vi "build_queue.vi"(8 "Scan settings array":T2[](array[typedef]) {"Settling delay (s)" min=0.0; "J-t illumination" items=["Light only", "Dark only", "Light then dark", "Dark then light"]; "Measurement speed" items=["Fast", "Normal", "High accuracy"]; "Illumination" items=["Light only", "Dark only", "Light then dark", "Dark then light"]; "Only repeat for best pixel" items=["only for best pixel", "for best 2 pixels", "for best 3 pixels", "for best 4 pixels", "for best 5 pixels", "for best 6 pixels", "for best 7 pixels", "for all pixels"]; "No. of repeat scans" min=1.0 step=1.0; "Max power best pixel only" items=["only the best pixel", "the best 2 pixels", "the best 3 pixels", "the best 4 pixels", "the best 5 pixels", "the best 6 pixels", "the best 7 pixels", "all pixels"]; "J-t best pixel only" items=["only the best pixel", "the best 2 pixels", "the best 3 pixels", "the best 4 pixels", "the best 5 pixels", "the best 6 pixels", "the best 7 pixels", "all pixels"]; "J-t measurement speed" items=["Fast", "Normal", "High Accuracy"]; "Stabilisation mode" items=["V", "I"]; "Measurement delay (s)" min=0.01}, 11 "Device details":T1={"Cell Position"=1, "Cell Label"="", "Pixel to measure"=0, "Area (cm^2)"=0.0919, "Variable"="", "Variable value"="", "Scan settings"=0} {"Scan settings" items=["Default_inv", "Default_std"]; "Pixel to measure" items=["All", "1", "2", "3", "4", "5", "6", "7", "8"]}) -> (3 "Measurement queue":T3(array[cluster]) {"Pixel to measure" items=["All", "1", "2", "3", "4", "5", "6", "7", "8"]})   [LabVIEW 2016]
uses:
  TypeDefs/scan_settings.ctl
panel:
  out "Max power best pixel only":u16
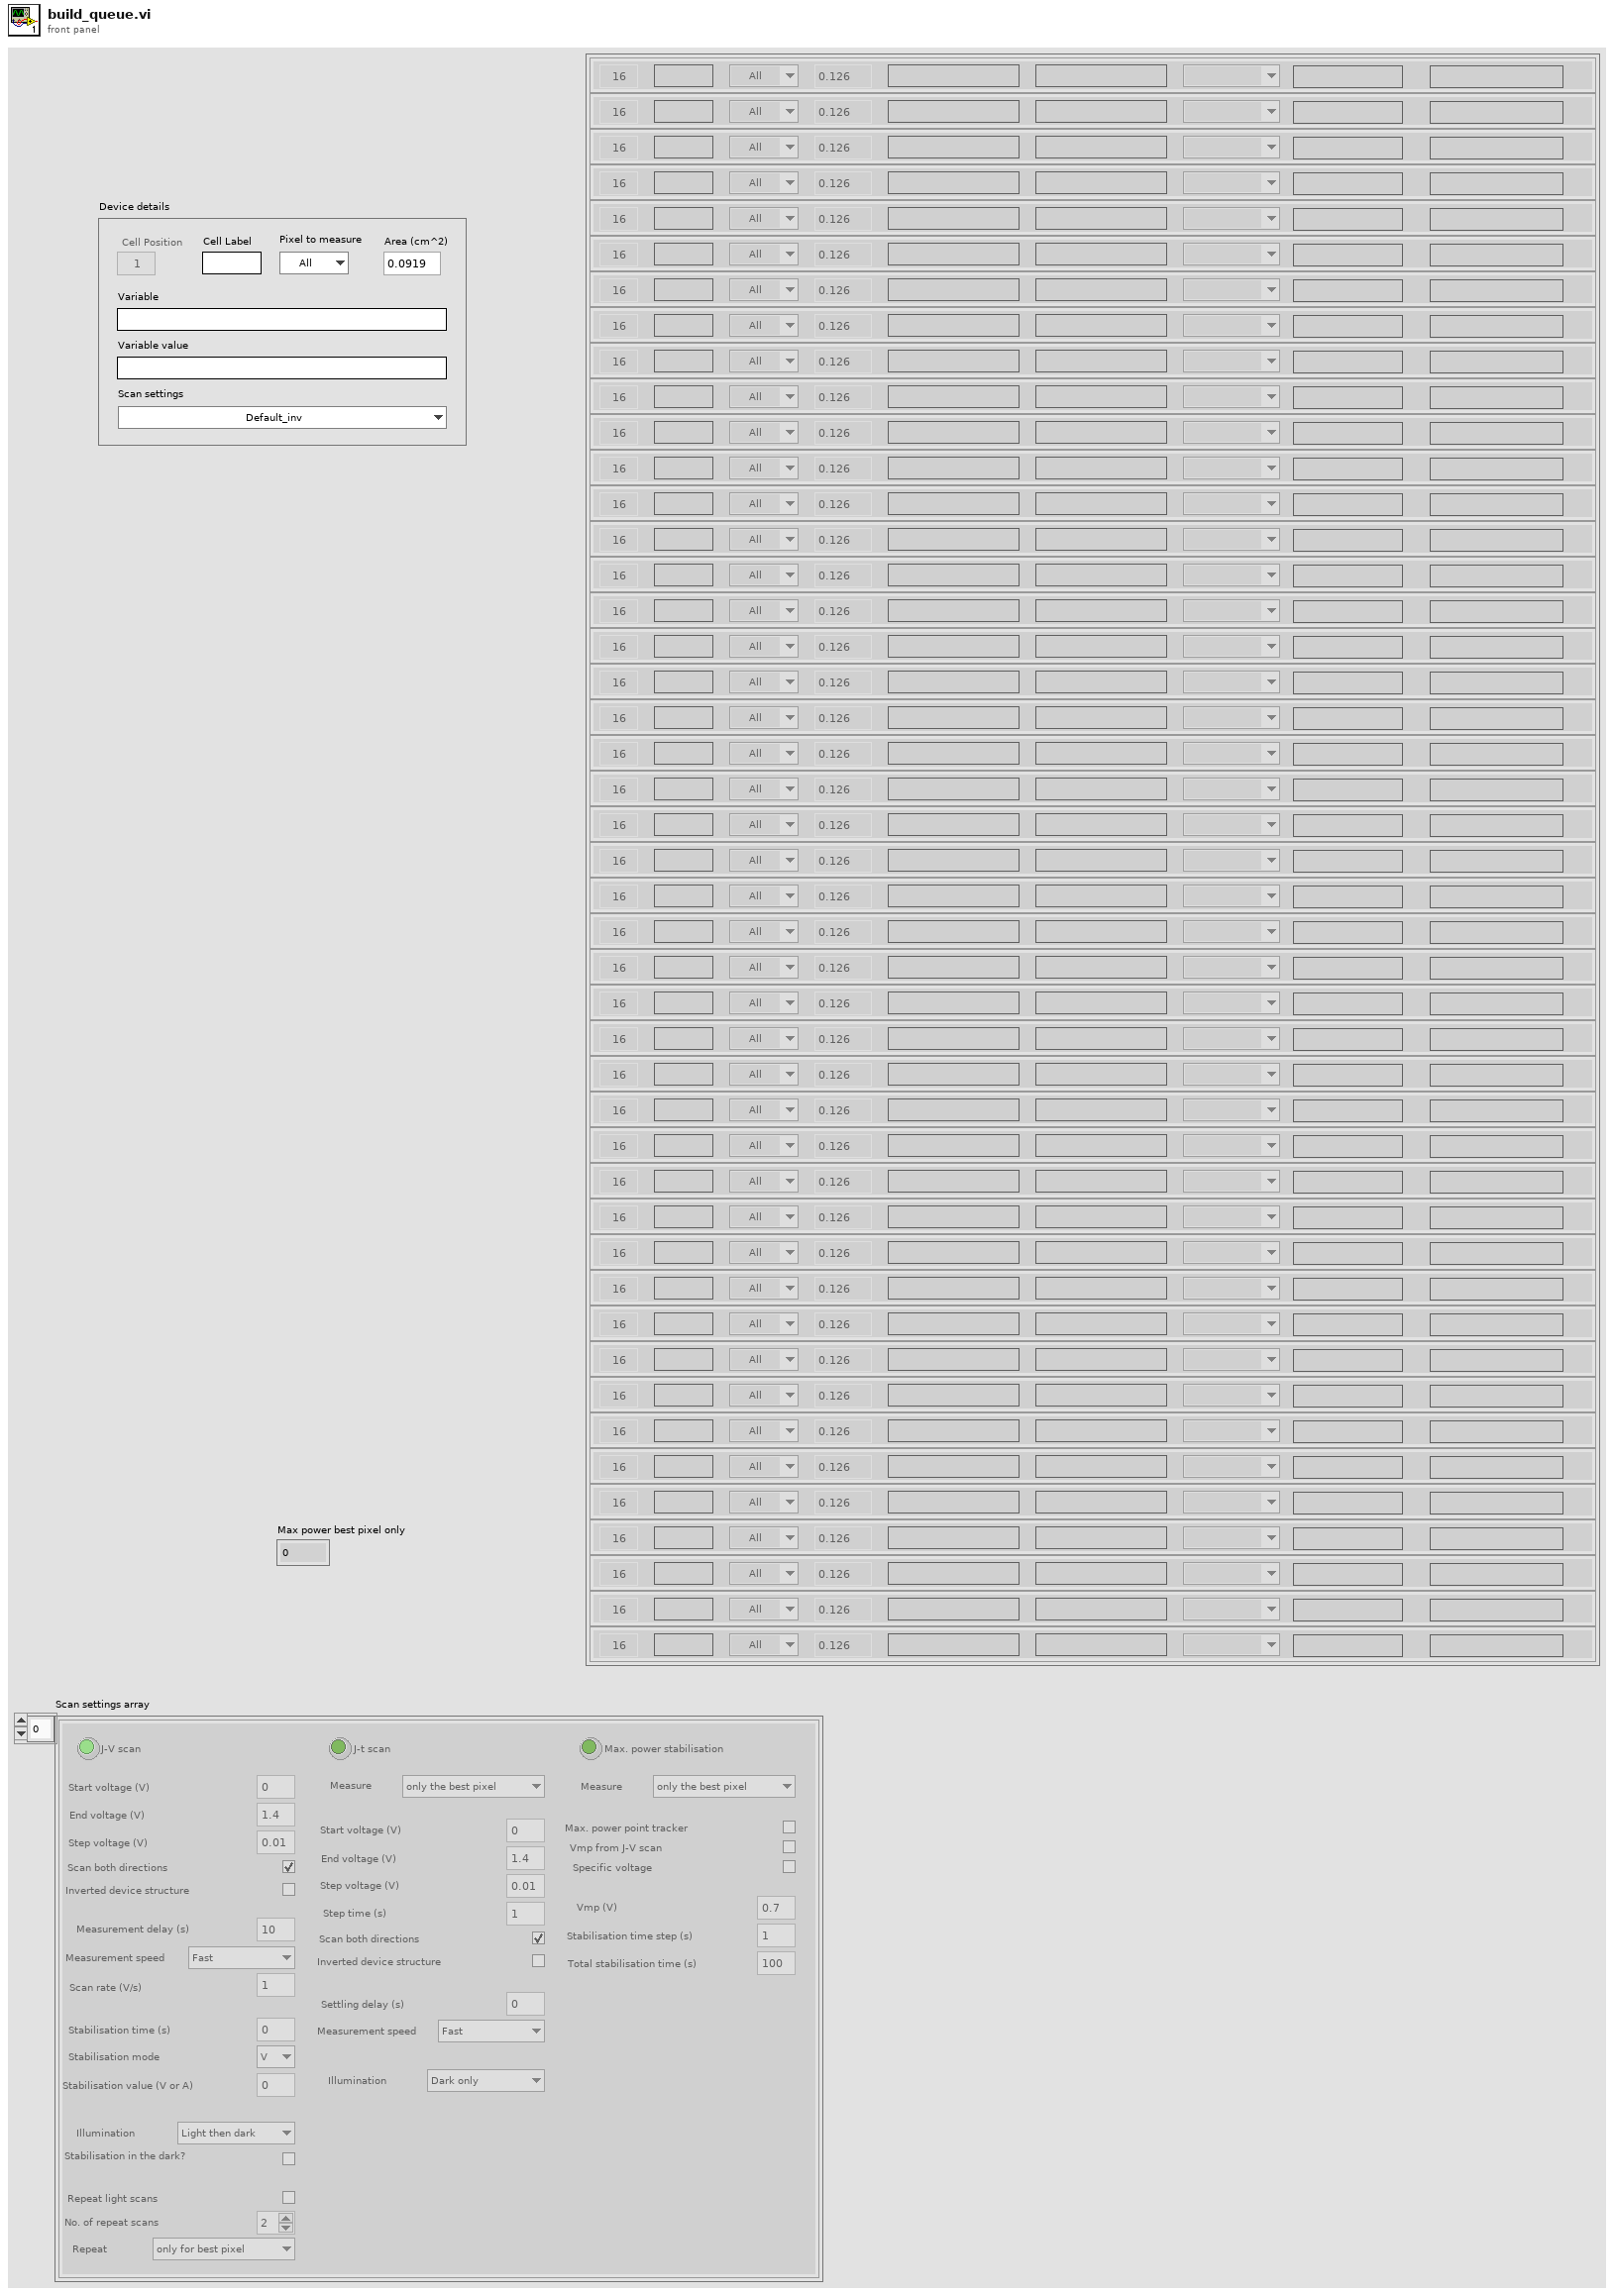
[diagram p1: front panel]
types:
  T1 = cluster{"Cell Position":i32, "Cell Label":string, "Pixel to measure":u16, "Area (cm^2)":dbl, "Variable":string, "Variable value":string, "Scan settings":u16}
  T2 = typedef "scan_settings.ctl" = cluster{"J-V scan":bool, "Start voltage (V)":dbl, "End voltage (V)":dbl, "Step voltage (V)":dbl, "Scan both directions":bool, "Inverted device structure":bool, "Measurement delay (s)":dbl, "Measurement speed":u8, "Scan rate (V/s)":dbl, "Stabilisation time (s)":dbl, "Stabilisation mode":u16, "Stabilisation value (V or A) ":dbl, "Illumination":u16, "Stabilisation in the dark?":bool, "Repeat light scans":bool, "No. of repeat scans":dbl, "Only repeat for best pixel":u16, "J-t scan":bool, "J-t best pixel only":u16, "J-t start voltage (V)":dbl, "J-t end voltage (V)":dbl, "J-t step voltage (V)":dbl, "Step time (s)":dbl, "J-t scan both directions":bool, "J-t inverted device structure":bool, "Settling delay (s)":dbl, "J-t measurement speed":u16, "J-t illumination":u16, "Max. power stabilisation":bool, "Max power best pixel only":u16, "Max. power point tracker":bool, "Vmp from J-V scan":bool, "Max P stab. Specific voltage":bool, "Vmp (V)":dbl, "Stabilisation time step (s)":dbl, "Total stabilisation time (s)":dbl}
  T3 = cluster{"Cell Position":i32, "Cell Label":string, "Pixel to measure":u16, "Area (cm^2)":dbl, "Variable":string, "Variable value":string, "Scan settings in queue":u16, "Light or dark":string, "Measurement type":string}[]
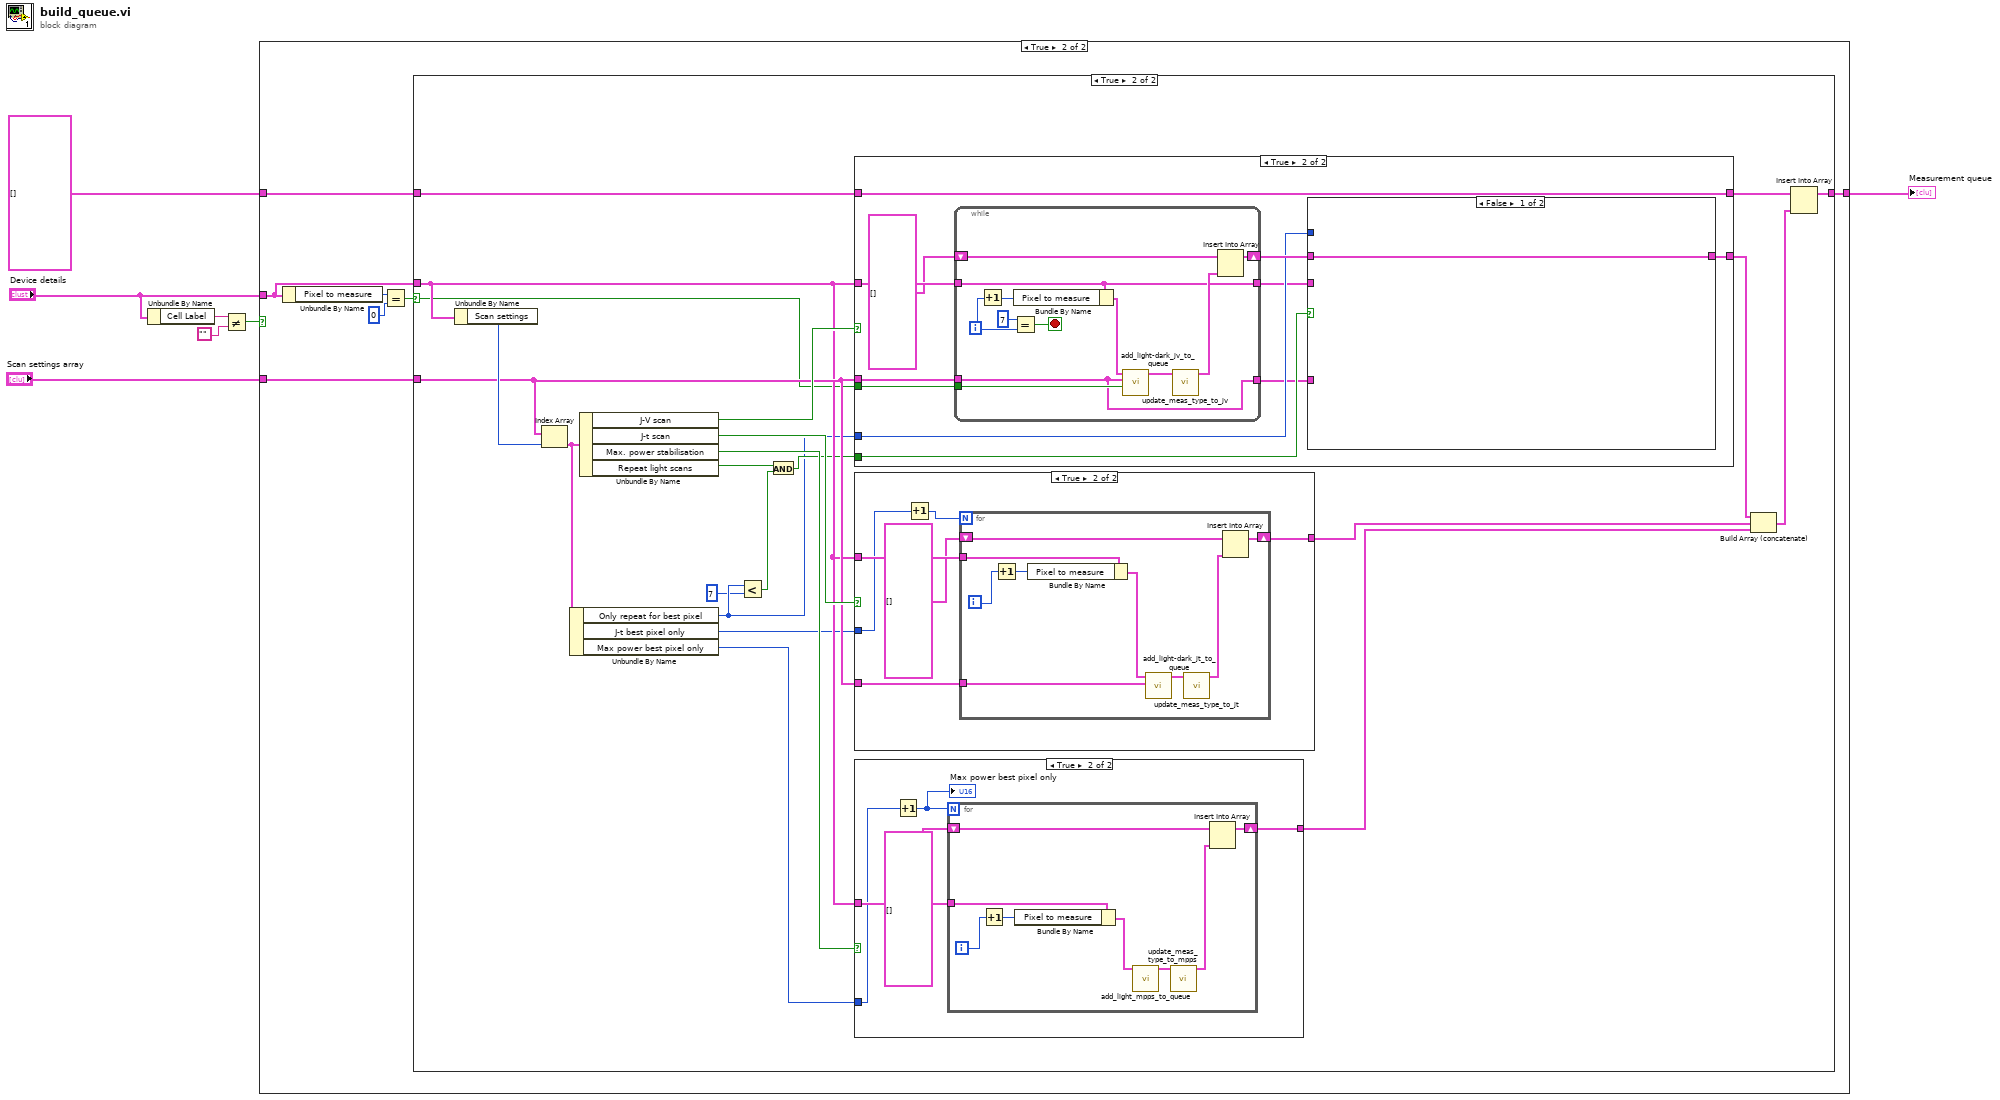
[diagram p0: block diagram]
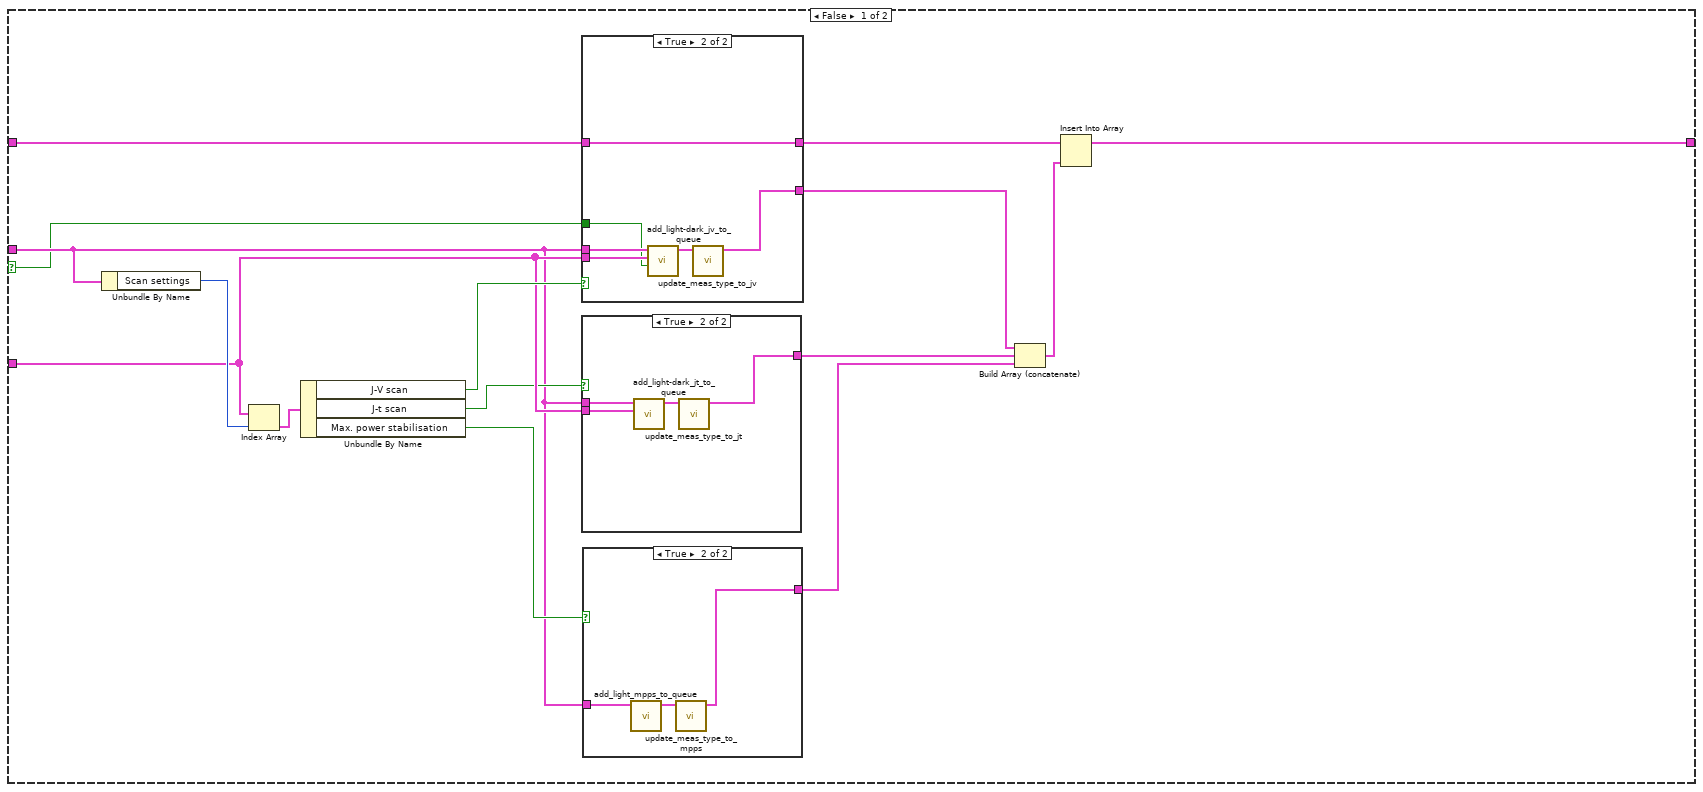
[diagram p3: hidden frame]
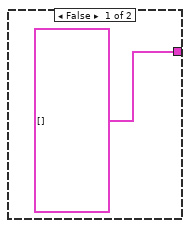
[diagram p4: hidden frame]
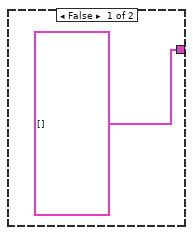
[diagram p5: hidden frame]
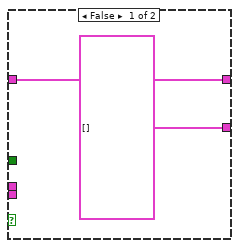
[diagram p6: hidden frame]
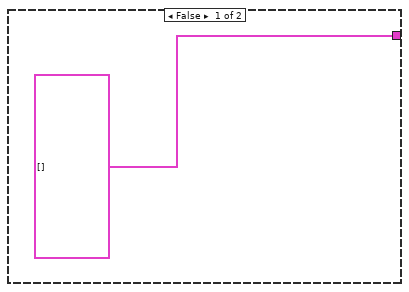
[diagram p7: hidden frame]
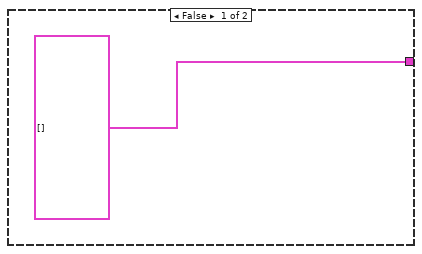
[diagram p8: hidden frame]
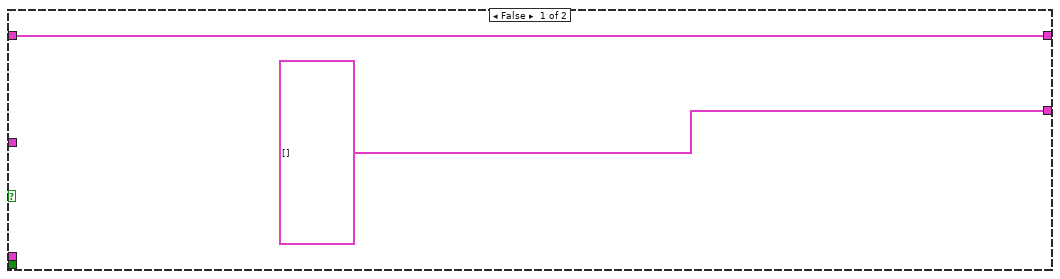
[diagram p9: hidden frame]
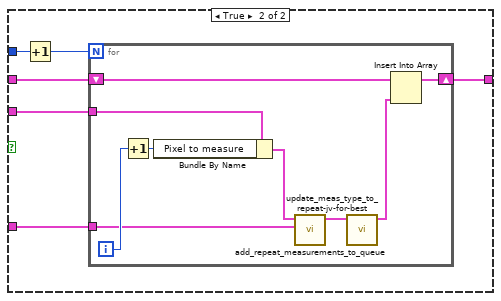
[diagram p10: hidden frame]
diagram:
  n1 = Unbundle By Name("Device details") -> ("Cell Label"=w3:string)
  n2 = Not Equal?(x=w3, y="") -> (x != y?=w1:bool)
  n3 = case shown="True" w1 {
    tunnel: [w8 w12] -> w6
    tunnel: "Device details" -> [_ w11]
    tunnel: T3 [] ("Measurement queue") -> [w8 w10]
    tunnel: "Scan settings array" -> [_ w9]
    frame False {
    }
    frame True {
      n4 = Unbundle By Name(w11) -> ("Pixel to measure"=w15:u16)
      n5 = Equal?(x=w15, y=0) -> (x = y?=w13:bool)
      n6 = case shown="True" w13 {
        selector: w13 -> [w16 w53]
        tunnel: w11 -> [w19 w60]
        tunnel: [w30 w67] -> w12
        tunnel: w10 -> [w20 w59]
        tunnel: w9 -> [w26 w63]
        frame False {
          n7 = Unbundle By Name(w19) -> ("Scan settings"=w29:u16)
          n8 = Index Array(array=w26, index=w29) -> (element=w18:T2)
          n9 = Unbundle By Name(w18) -> ("J-V scan"=w27:bool, "J-t scan"=w25:bool, "Max. power stabilisation"=w21:bool)
          n10 = case shown="True" w27 {
            tunnel: w19 -> [_ w46]
            tunnel: w26 -> [_ w45]
            tunnel: [w41 w44] -> w28
            tunnel: w20 -> [w41 w44]
            tunnel: [T3 [] ("Measurement queue") w43] -> w17
            tunnel: w16 -> [_ w42]
            frame False {
            }
            frame True {
              n11 = call "add_light-dark_jv_to_queue.vi"("Measuring all pixels on cell?"=w42, "Scan settings array"=w45, "Cell settings cluster"=w46) -> ("Light/dark array"=w47:T3)  [unwired: 8 in]
              n12 = call "update_meas_type_to_jv.vi"("Cell details array in"=w47) -> ("Cell details array out"=w43:T3)  [unwired: 10 in]
            }
          }
          n13 = case shown="True" w25 {
            tunnel: w19 -> [_ w38]
            tunnel: w26 -> [_ w37]
            tunnel: [T3 [] ("Measurement queue") w36] -> w24
            frame False {
            }
            frame True {
              n14 = call "add_light-dark_jt_to_queue.vi"("Scan settings array"=w37, "Cell settings cluster"=w38) -> ("Light/dark array"=w39:T3)  [unwired: 9 in]
              n15 = call "update_meas_type_to_jt.vi"("Cell details array in"=w39) -> ("Cell details array out"=w36:T3)  [unwired: 10 in]
            }
          }
          n16 = case shown="True" w21 {
            tunnel: [T3 [] ("Measurement queue") w32] -> w23
            tunnel: w19 -> [_ w33]
            frame False {
            }
            frame True {
              n17 = call "add_light_mpps_to_queue.vi"("Cell settings cluster"=w33) -> ("Light/dark array"=w34:T3)  [unwired: 10 in]
              n18 = call "update_meas_type_to_mpps.vi"("Cell details array in"=w34) -> ("Cell details array out"=w32:T3)  [unwired: 10 in]
            }
          }
          n19 = Build Array (concatenate)(w17, w24, w23) -> (w22:T3)
          n20 = Insert Into Array(array=w28, new element=w22) -> (w30:T3)  [unwired: 1 in]
        }
        frame True {
          n21 = Unbundle By Name(w60) -> ("Scan settings"=w69:u16)
          n22 = Index Array(array=w63, index=w69) -> (element=w56:T2)
          n23 = Unbundle By Name(w56) -> ("Only repeat for best pixel"=w49:u16, "J-t best pixel only"=w55:u16, "Max power best pixel only"=w54:u16)
          n24 = Unbundle By Name(w56) -> ("J-V scan"=w68:bool, "J-t scan"=w64:bool, "Max. power stabilisation"=w62:bool, "Repeat light scans"=w52:bool)
          n25 = Less?(x=w49, y=u16 7 ("x")) -> (x < y?=w51:bool)
          n26 = And(x=w52, y=w51) -> (x .and. y?=w50:bool)
          n27 = case shown="True" w68 {
            tunnel: [w101 w110] -> w58
            tunnel: w59 -> [w101 w110]
            tunnel: w60 -> [_ w112]
            tunnel: w63 -> [_ w111]
            tunnel: [T3 [] ("Measurement queue") w108] -> w57
            tunnel: w53 -> [_ w109]
            tunnel: w50 -> [_ w106]
            tunnel: w49 -> [_ w105]
            frame False {
            }
            frame True {
              n28 = while {
                tunnel: w112 -> [w114]
                shift-right: [w120] -> w107
                shift-left: T3 [] ("Measurement queue") -> [w119]
                tunnel: w111 -> [w113]
                tunnel: w109 -> [w115]
                tunnel: [w114] -> w104
                tunnel: [w113] -> w103
                i -> [w122]
                stop <- w124 stop-if-true
                n29 = Increment(x=w122) -> (x+1=w123:i32)
                n30 = Equal?(x=7, y=w122) -> (x = y?=w124:bool)
                n31 = Bundle By Name(cluster=w114, "Pixel to measure"=w123) -> (w118:T1)
                n32 = call "add_light-dark_jv_to_queue.vi"("Measuring all pixels on cell?"=w115, "Scan settings array"=w113, "Cell settings cluster"=w118) -> ("Light/dark array"=w117:T3)  [unwired: 8 in]
                n33 = call "update_meas_type_to_jv.vi"("Cell details array in"=w117) -> ("Cell details array out"=w116:T3)  [unwired: 10 in]
                n34 = Insert Into Array(array=w119, new element=w116) -> (w120:T3)  [unwired: 1 in]
              }
              n35 = case shown="False" w106 {
                tunnel: [w125 w130] -> w108
                tunnel: w107 -> [w125 w131]
                tunnel: w105 -> [_ w127]
                tunnel: w104 -> [_ w129]
                tunnel: w103 -> [_ w128]
                frame False {
                }
                frame True {
                  n36 = Increment(x=w127) -> (x+1=w126:u16)
                  n37 = for {
                    N: w126 -> [_]
                    shift-right: [w139] -> w130
                    shift-left: w131 -> [w140]
                    tunnel: w129 -> [w134]
                    tunnel: w128 -> [w133]
                    i -> [w138]
                    n38 = Increment(x=w138) -> (x+1=w137:i32)
                    n39 = Bundle By Name(cluster=w134, "Pixel to measure"=w137) -> (w136:T1)
                    n40 = call "add_repeat_measurements_to_queue.vi"("Scan settings array"=w133, "Cell settings cluster"=w136) -> ("Repeat light array"=w135:T3)  [unwired: 9 in]
                    n41 = call "update_meas_type_to_repeat-jv-for-best.vi"("Cell details array in"=w135) -> ("Cell details array out"=w132:T3)  [unwired: 10 in]
                    n42 = Insert Into Array(array=w140, new element=w132) -> (w139:T3)  [unwired: 1 in]
                  }
                }
              }
            }
          }
          n43 = case shown="True" w64 {
            tunnel: [T3 [] ("Measurement queue") w90] -> w65
            tunnel: w60 -> [_ w89]
            tunnel: w63 -> [_ w88]
            tunnel: w55 -> [_ w85]
            frame False {
            }
            frame True {
              n44 = Increment(x=w85) -> (x+1=w86:u16)
              n45 = for {
                N: w86 -> [_]
                tunnel: w89 -> [w97]
                shift-right: [w96] -> w90
                shift-left: T3 [] ("Measurement queue") -> [w95]
                tunnel: w88 -> [w93]
                i -> [w98]
                n46 = Increment(x=w98) -> (x+1=w99:i32)
                n47 = Bundle By Name(cluster=w97, "Pixel to measure"=w99) -> (w94:T1)
                n48 = call "add_light-dark_jt_to_queue.vi"("Scan settings array"=w93, "Cell settings cluster"=w94) -> ("Light/dark array"=w92:T3)  [unwired: 9 in]
                n49 = call "update_meas_type_to_jt.vi"("Cell details array in"=w92) -> ("Cell details array out"=w91:T3)  [unwired: 10 in]
                n50 = Insert Into Array(array=w95, new element=w91) -> (w96:T3)  [unwired: 1 in]
              }
            }
          }
          n51 = case shown="True" w62 {
            tunnel: [T3 [] ("Measurement queue") w75] -> w61
            tunnel: w60 -> [_ w74]
            tunnel: w54 -> [_ w72]
            frame False {
            }
            frame True {
              n52 = Increment(x=w72) -> (x+1=w71:u16)
              "Max power best pixel only" <- w71
              n53 = for {
                N: w71 -> [_]
                tunnel: w74 -> [w81]
                shift-right: [w80] -> w75
                shift-left: T3 [] ("Measurement queue") -> [w79]
                i -> [w82]
                n54 = Increment(x=w82) -> (x+1=w83:i32)
                n55 = Bundle By Name(cluster=w81, "Pixel to measure"=w83) -> (w78:T1)
                n56 = call "add_light_mpps_to_queue.vi"("Cell settings cluster"=w78) -> ("Light/dark array"=w77:T3)  [unwired: 10 in]
                n57 = call "update_meas_type_to_mpps.vi"("Cell details array in"=w77) -> ("Cell details array out"=w76:T3)  [unwired: 10 in]
                n58 = Insert Into Array(array=w79, new element=w76) -> (w80:T3)  [unwired: 1 in]
              }
            }
          }
          n59 = Build Array (concatenate)(w57, w65, w61) -> (w66:T3)
          n60 = Insert Into Array(array=w58, new element=w66) -> (w67:T3)  [unwired: 1 in]
        }
      }
    }
  }
  "Measurement queue" <- w6
